vi "Layout Table.vi"(0 "Listbox Ref":refnum<vi>, 9 "Columns":T1[](array[typedef]), 12 "row headers":bool) -> (4 "reference out":refnum<vi>)   [LabVIEW 2015, in "KTable.xctl"]
uses:
  KTable.xctl
  ColumnSpec.ctl
  ColumnType.ctl
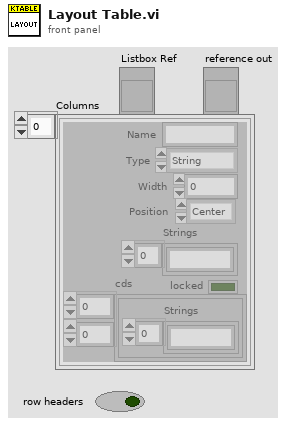
[diagram p1: front panel]
types:
  T1 = typedef "KTable.xctl/ColumnSpec.ctl" = cluster{"Name":string, "Type":T2, "Width":i32, "Strings":string[], "Position":enum16{"Left", "Center", "Right"}, "locked":bool, "cds":cluster{"Strings":string[]}[][]}
  T2 = typedef "KTable.xctl/ColumnType.ctl" = enum16{"String", "Enum", "Int", "Double", "Boolean", "Ring", "Formula", "Color"}
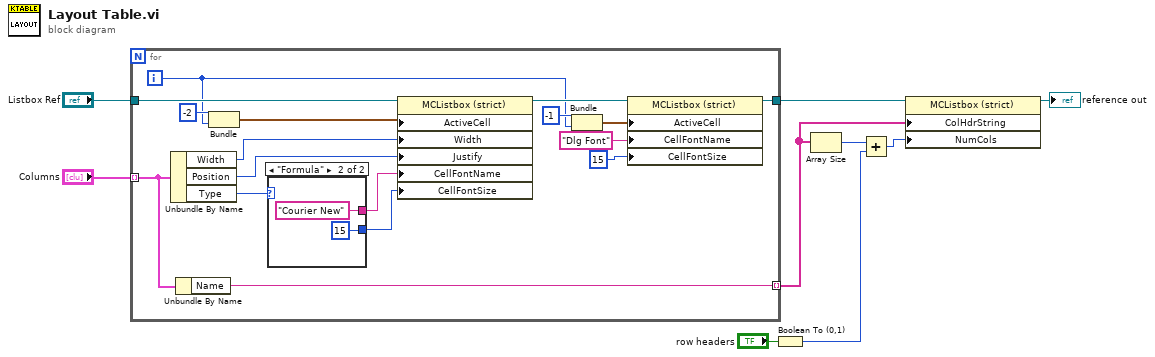
[diagram p0: block diagram]
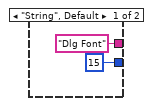
[diagram p2: hidden frame]
diagram:
  n1 = for {
    tunnel: "Columns" -> [w22] mode=indexing
    tunnel: [w21] -> w7 mode=indexing
    tunnel: "Listbox Ref" -> [w26]
    tunnel: [w15] -> w6
    i -> [w10]
    n2 = Unbundle By Name(w22) -> ("Width"=w23:i32, "Position"=w20:enum16{"Left", "Center", "Right"}, "Type"=w19:T2)
    n3 = Unbundle By Name(w22) -> ("Name"=w21:string)
    n4 = Bundle(-2, w10) -> (w24:cluster{i32, i32})  [unwired: 1 in]
    n5 = case shown="\"Formula\"" w19 {
      tunnel: ["Dlg Font" ("Active Cell:Cell Font:Name") "Courier New" ("Active Cell:Cell Font:Name")] -> w18
      tunnel: [u32 15 ("Active Cell:Cell Font:Size") u32 15 ("Active Cell:Cell Font:Size")] -> w17
      frame "String", Default {
      }
      frame "Formula" {
      }
    }
    n6 = property class="MCListbox (strict)"(reference=w26, "ActiveCell"=w24, "Width"=w23, "Justify"=w20, "CellFontName"=w18, "CellFontSize"=w17) -> (reference out=w16:refnum<vi>)  [unwired: 1 in, 1 out]
    n7 = Bundle(-1, w10) -> (w11:cluster{i32, i32})  [unwired: 1 in]
    n8 = property class="MCListbox (strict)"(reference=w16, "ActiveCell"=w11, "CellFontName"="Dlg Font" ("Active Cell:Cell Font:Name"), "CellFontSize"=u32 15 ("Active Cell:Cell Font:Size")) -> (reference out=w15:refnum<vi>)  [unwired: 1 in, 1 out]
  }
  n9 = Boolean To (0,1)(Boolean="row headers") -> (0, 1=w2:i16)
  n10 = Array Size(array=w7) -> (size(s)=w8:i32)
  n11 = Add(x=w8, y=w2) -> (x+y=w1:i32)
  n12 = property class="MCListbox (strict)"(reference=w6, "ColHdrString"=w7, "NumCols"=w1) -> (reference out=→"reference out":refnum<vi>)  [unwired: 1 in, 1 out]
